vi "MakePaths.vi"(10 "number":i32, 11 "Path":path) -> (1 "BIN":path, 2 "TDMS":path, 3 "AVI":path)   [LabVIEW 2013]
panel:
  in  "String":string
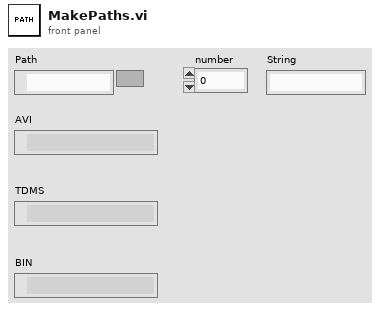
[diagram p1: front panel]
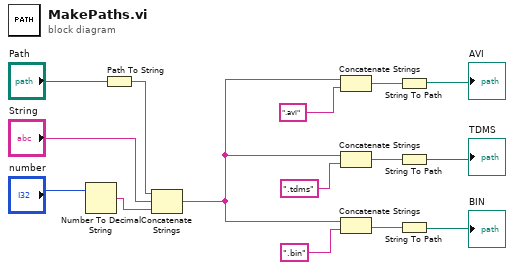
[diagram p0: block diagram]
diagram:
  n1 = Number To Decimal String(number="number") -> (decimal integer string=w14:string)  [unwired: 1 in]
  n2 = Path To String(path="Path") -> (string=w9:string)
  n3 = Concatenate Strings(w9, "String", w14) -> (w3:string)
  n4 = Concatenate Strings(w3, ".avi" ("name")) -> (w7:string)
  n5 = Concatenate Strings(w3, ".tdms" ("name")) -> (w6:string)
  n6 = Concatenate Strings(w3, ".bin" ("name")) -> (w2:string)
  n7 = String To Path(string=w7) -> (path=→"AVI":path)
  n8 = String To Path(string=w6) -> (path=→"TDMS":path)
  n9 = String To Path(string=w2) -> (path=→"BIN":path)
